vi "Show Nested Panel.vi"(8 "error in":errorcluster, 10 "Panel Ident":string, 11 "Study Actor in":refnum<class "Study Actor.lvclass">) -> (0 "error out":errorcluster, 3 "Study Actor out":refnum<class "Study Actor.lvclass">)   [LabVIEW 2023, in "HAL GOOP4.lvlib" / "Study Actor.lvlib" / "Study Actor.lvclass"]
uses:
  Study Actor.lvclass
  <vilib>/MGI/Panel Manager/Panel Actor/Panel Actor Messages/Show Panel Msg/Show Panel Msg.lvclass
  <vilib>/ErrorRing/Error Ring.xnode
  <vilib>/Utility/error.llb/Error Cluster From Error Code.vi
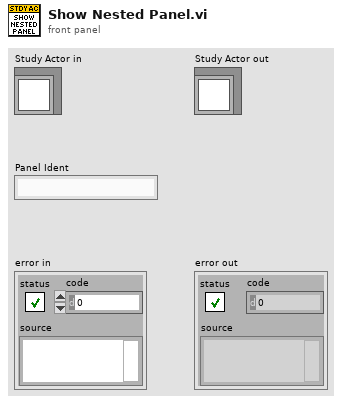
[diagram p1: front panel]
types:
  T1 = map{string, refnum<class "Message Enqueuer.lvclass">}
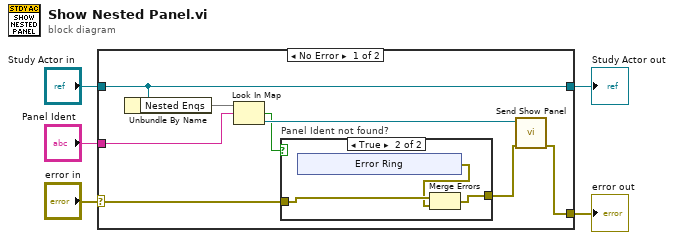
[diagram p0: block diagram]
diagram:
  n1 = case shown="No Error" "error in" {
    selector: "error in" -> [w8 w24]
    tunnel: [w6 w24] -> w4
    tunnel: [w13 w23] -> w2
    tunnel: "Study Actor in" -> [w13 w23]
    tunnel: "Panel Ident" -> [w11 _]
    frame No Error {
      n2 = Unbundle By Name(w13) -> ("Nested Enqs"=w12:T1)
      n3 = Look In Map(map=w12, key=w11) -> (key not found?=w9:bool, value=w10:refnum<class "Message Enqueuer.lvclass">)  [unwired: 1 in]
      n4 = case "Panel Ident not found?" shown="True" w9 {
        tunnel: w8 -> [w14 w17]
        tunnel: [w14 w15] -> w7
        frame False {
        }
        frame True {
          n5 = xnode "Error Ring"() -> ("error out"=w16:errorcluster)
          n6 = Merge Errors(w17, w16) -> (w15:errorcluster)
        }
      }
      n7 = call <vilib>:"Send Show Panel.vi"("Error In"=w7, "Message Enqueuer in"=w10) -> ("Error Out"=w6:errorcluster)  [unwired: 8 in, 1 out]
    }
    frame Error {
    }
  }
  "error out" <- w4
  "Study Actor out" <- w2
